vi "StringWeb.vi"(8 "错误输入":errorcluster, 9 "value":string, 10 "string in":string, 11 "refnum in":refnum<k7>) -> (0 "错误输出":errorcluster, 3 "refnum out":refnum<k7>)   [LabVIEW 2013]
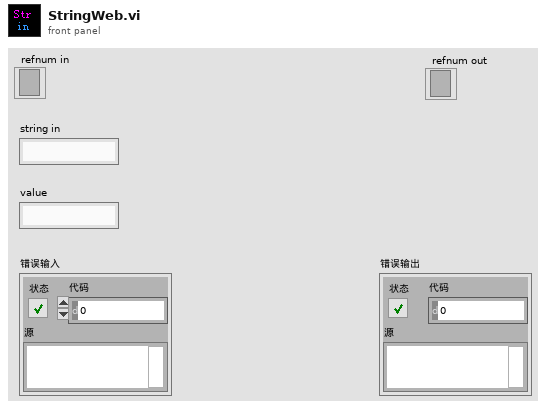
[diagram p1: front panel]
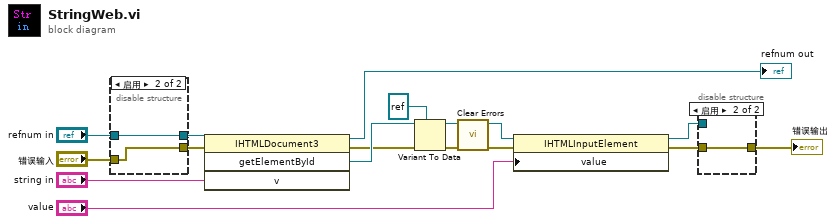
[diagram p0: block diagram]
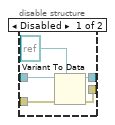
[diagram p2: hidden frame]
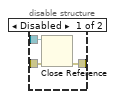
[diagram p3: hidden frame]
diagram:
  n1 = disable-structure shown="启用" {
    disable-tunnel: [w20 w23] -> w16
    disable-tunnel: "refnum in" -> [w19 w23]
    disable-tunnel: "错误输入" -> [w18 w22]
    disable-tunnel: [w17 w22] -> w3
    frame Disabled {
      n2 = Variant To Data(error in=w18, type=refnum<k7> refnum ("引用输出"), Variant=w19) -> (data=w20:refnum<k7>, error out=w17:errorcluster)
    }
    frame Enabled {
    }
  }
  n3 = invoke on="调用节点" class="IHTMLDocument3" method="getElementById"(reference=w16, error in=w3, "v"="string in") -> (reference out=→"refnum out":refnum<k7>, error out=w7:errorcluster, "getElementById"=w12:refnum<k7>)  [unwired: 1 in, 1 out]
  n4 = Variant To Data(error in=w7, type=refnum<k7> refnum ("引用输出"), Variant=w12) -> (data=w13:refnum<k7>, error out=w6:errorcluster)
  n5 = call <vilib>:"Clear Errors.vi"("error in (no error)"=w6) -> ("error out"=w1:errorcluster)  [unwired: 6 in]
  n6 = property on="属性节点" class="IHTMLInputElement"(reference=w13, error in=w1, "value"="value") -> (reference out=w9:refnum<k7>, error out=w8:errorcluster)
  n7 = disable-structure shown="启用" {
    disable-tunnel: w9 -> [w26 _]
    disable-tunnel: w8 -> [w25 w27]
    disable-tunnel: [w24 w27] -> w5
    frame Disabled {
      n8 = Close Reference(reference=w26, error in (no error)=w25) -> (error out=w24:errorcluster)
    }
    frame Enabled {
    }
  }
  "错误输出" <- w5
